vi "Get State.vi"(8 "error in (no error)":errorcluster, 11 "Keithley 622x2182 Driver in":refnum<class "Keithley 622x2182 Driver.lvclass">) -> (0 "error out":errorcluster, 1 "Data ready":bool, 2 "Armed":bool, 3 "Keithley 622x2182 Driver out":refnum<class "Keithley 622x2182 Driver.lvclass">, 4 "Availiable Samples":u32, 5 "Finished":bool)   [LabVIEW 2021, in "Keithley 622x2182 Driver.lvclass"]
uses:
  Keithley 622x2182 Driver.lvclass
  C:/Git/NHMFL_Core/Libraries/Instruments/VISA Instrument/VISA Instrument.lvclass
  VISA Instrument/VISA Instrument.lvclass/VISA Instrument.ctl
  VISA Instrument/Read VISA resource.vi
  VISA Instrument/Write VISA resource.vi
panel:
  out "read buffer 2":string
  out "General Settings:Timeout Value":u32
  out "read buffer":string
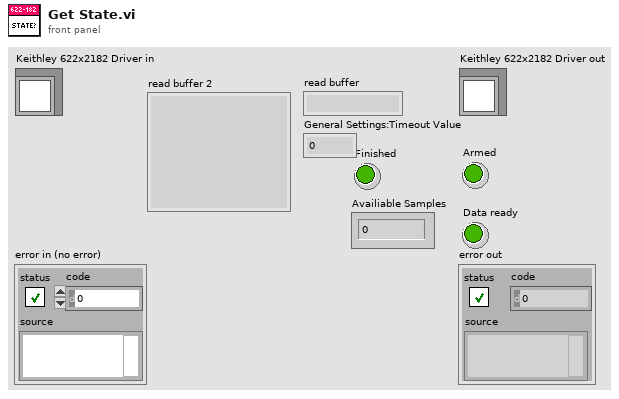
[diagram p1: front panel]
types:
  T1 = typedef "Stepper Config.ctl" = cluster{"Start":dbl, "End":dbl, "Step":dbl, "Scan shape":enum16{"Sawtooth", "Triangular"}, "Append measurements":string[]}
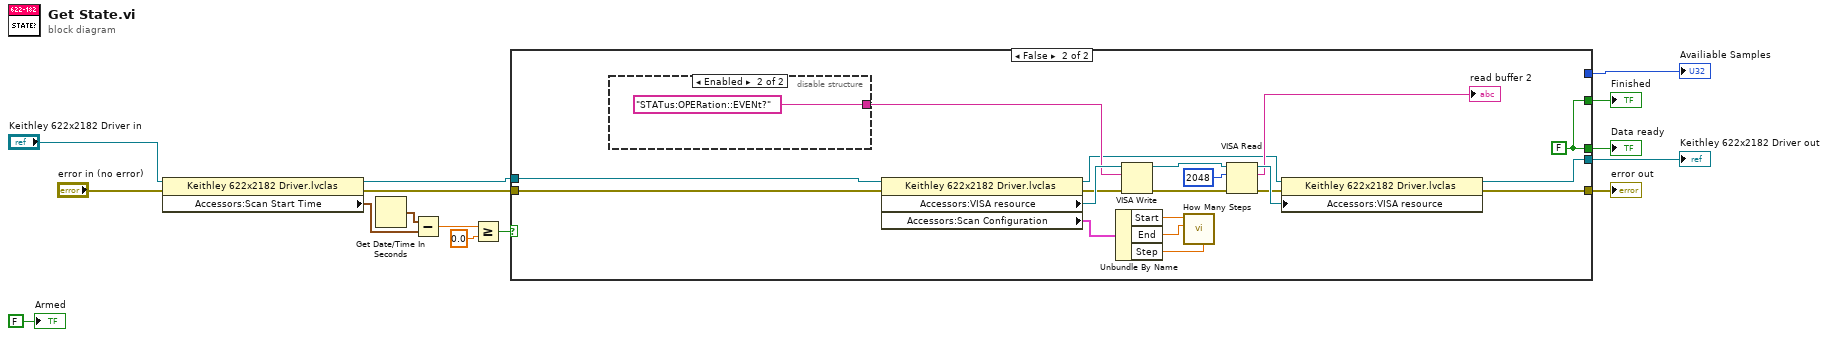
[diagram p0: block diagram]
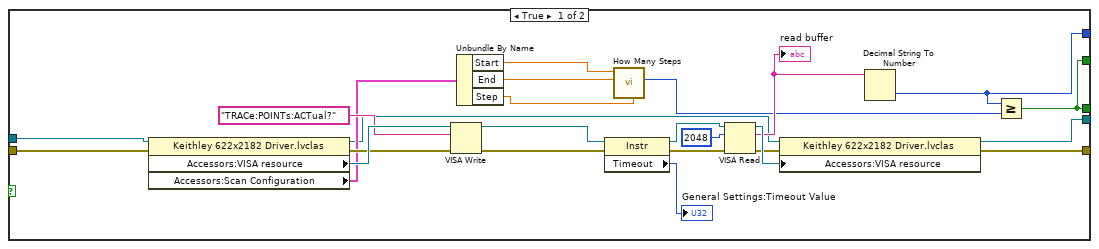
[diagram p2: hidden frame]
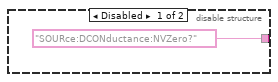
[diagram p3: hidden frame]
diagram:
  n1 = property class="Keithley 622x2182 Driver.lvclas"(reference="Keithley 622x2182 Driver in", error in="error in (no error)") -> (reference out=w8:refnum<class "Keithley 622x2182 Driver.lvclass">, error out=w10:errorcluster, "Accessors:Scan Start Time"=w6:timestamp)
  n2 = Get Date/Time In Seconds() -> (seconds since 1Jan1904=w7:timestamp)
  n3 = Subtract(x=w7, y=w6) -> (x-y=w5:dbl)
  n4 = Greater Or Equal?(x=w5, y=0.0) -> (x >= y?=w3:bool)
  n5 = case shown="False" w3 {
    tunnel: [w32 w51] -> w15
    tunnel: [w31 w50] -> w13
    tunnel: [w16 w40] -> w2
    tunnel: [w24 _] -> w12
    tunnel: w10 -> [w18 w42]
    tunnel: w8 -> [w17 w41]
    tunnel: [w16 w40] -> w1
    frame True {
      n6 = property class="Keithley 622x2182 Driver.lvclas"(reference=w17, error in=w18) -> (reference out=w23:refnum<class "Keithley 622x2182 Driver.lvclass">, error out=w38:errorcluster, "Accessors:VISA resource"=w39:refnum<visa-resource-name>, "Accessors:Scan Configuration"=w30:T1)
      n7 = VISA Write(VISA resource name=w39, write buffer="TRACe:POINTs:ACTual?", error in (no error)=w38) -> (VISA resource name out=w21:refnum<visa-resource-name>, error out=w36:errorcluster)  [unwired: 1 out]
      n8 = Unbundle By Name(w30) -> ("Start"=w29:dbl, "End"=w28:dbl, "Step"=w27:dbl)
      n9 = property class="Instr"(reference=w21, error in=w36) -> (reference out=w20:refnum<visa-resource-name>, error out=w22:errorcluster, "Timeout"=→"General Settings:Timeout Value":u32)
      n10 = call "How Many Steps.vi"("Step"=w27, "End"=w28, "Start"=w29) -> ("Number of steps out"=w25:i32)  [unwired: 6 in, 2 out]
      n11 = VISA Read(VISA resource name=w20, byte count=u32 2048, error in (no error)=w22) -> (VISA resource name out=w34:refnum<visa-resource-name>, read buffer=w26:string, error out=w33:errorcluster)  [unwired: 1 out]
      "read buffer" <- w26
      n12 = property class="Keithley 622x2182 Driver.lvclas"(reference=w23, error in=w33, "Accessors:VISA resource"=w34) -> (reference out=w32:refnum<class "Keithley 622x2182 Driver.lvclass">, error out=w31:errorcluster)
      n13 = Decimal String To Number(string=w26) -> (number=w24:i32)  [unwired: 2 in, 1 out]
      n14 = Greater Or Equal?(x=w24, y=w25) -> (x >= y?=w16:bool)
    }
    frame False {
      w40 = FALSE
      n15 = disable-structure shown="Enabled" {
        disable-tunnel: ["SOURce:DCONductance:NVZero?" "STATus:OPERation::EVENt?"] -> w56
        frame Disabled {
        }
        frame Enabled {
        }
      }
      n16 = property class="Keithley 622x2182 Driver.lvclas"(reference=w41, error in=w42) -> (reference out=w44:refnum<class "Keithley 622x2182 Driver.lvclass">, error out=w57:errorcluster, "Accessors:VISA resource"=w58:refnum<visa-resource-name>, "Accessors:Scan Configuration"=w49:T1)
      n17 = Unbundle By Name(w49) -> ("Start"=w48:dbl, "End"=w47:dbl, "Step"=w46:dbl)
      n18 = VISA Write(VISA resource name=w58, write buffer=w56, error in (no error)=w57) -> (VISA resource name out=w43:refnum<visa-resource-name>, error out=w55:errorcluster)  [unwired: 1 out]
      n19 = call "How Many Steps.vi"("Step"=w46, "End"=w47, "Start"=w48) -> ()  [unwired: 6 in, 3 out]
      n20 = VISA Read(VISA resource name=w43, byte count=u32 2048, error in (no error)=w55) -> (VISA resource name out=w53:refnum<visa-resource-name>, read buffer=→"read buffer 2":string, error out=w52:errorcluster)  [unwired: 1 out]
      n21 = property class="Keithley 622x2182 Driver.lvclas"(reference=w44, error in=w52, "Accessors:VISA resource"=w53) -> (reference out=w51:refnum<class "Keithley 622x2182 Driver.lvclass">, error out=w50:errorcluster)
    }
  }
  "error out" <- w13
  "Keithley 622x2182 Driver out" <- w15
  "Availiable Samples" <- w12
  "Finished" <- w1
  "Data ready" <- w2
  "Armed" <- FALSE ("Armed")
